vi "humedad.vi"(9 "error in (no error)":errorcluster, 10 "COM Bluegiga in":refnum<visa-resource-name>) -> (0 "error out":errorcluster, 2 "Text":string caption="Result", 3 "COM Bluegiga out":refnum<visa-resource-name>)   [LabVIEW 2020]
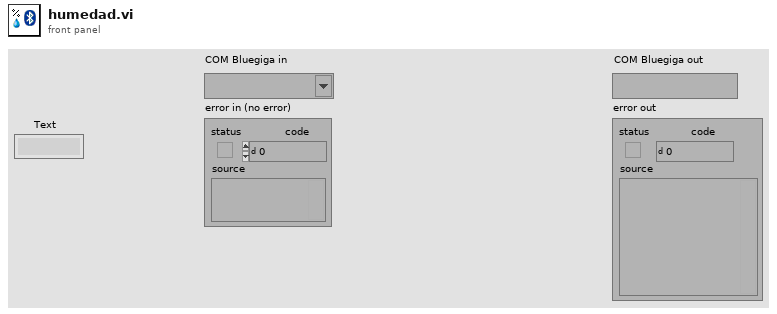
[diagram p1: front panel]
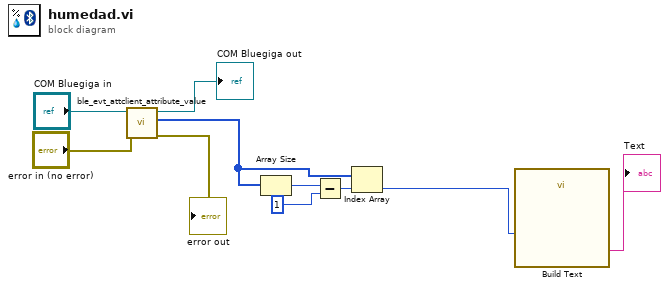
[diagram p0: block diagram]
diagram:
  n1 = call <vilib>:"ble_evt_attclient_attribute_value.vi"("error in (no error)"="error in (no error)", "COM Bluegiga in"="COM Bluegiga in") -> ("error out"=→"error out":errorcluster, "characteristic value"=w7:u8[], "COM Bluegiga out"=→"COM Bluegiga out":refnum<visa-resource-name>)  [unwired: 6 in, 1 out]
  n2 = Array Size(array=w7) -> (size(s)=w6:i32)
  n3 = Subtract(x=w6, y=1) -> (x-y=w9:i32)
  n4 = Index Array(array=w7, index=w9) -> (element=w1:u8)
  n5 = call "Build Text"("T"=w1) -> ("Result"=→"Text":string)  [unwired: 13 in, 1 out]
